vi "PrinterBarCode.vi"(8 "error in (no error)":errorcluster, 10 "PrintNum":u16 caption="列印數:", 11 "Data In":T1) -> (0 "error out":errorcluster, 3 "Data Out":T1)   [LabVIEW 2014]
uses:
  controls/Data1.ctl
  controls/Payjson.ctl
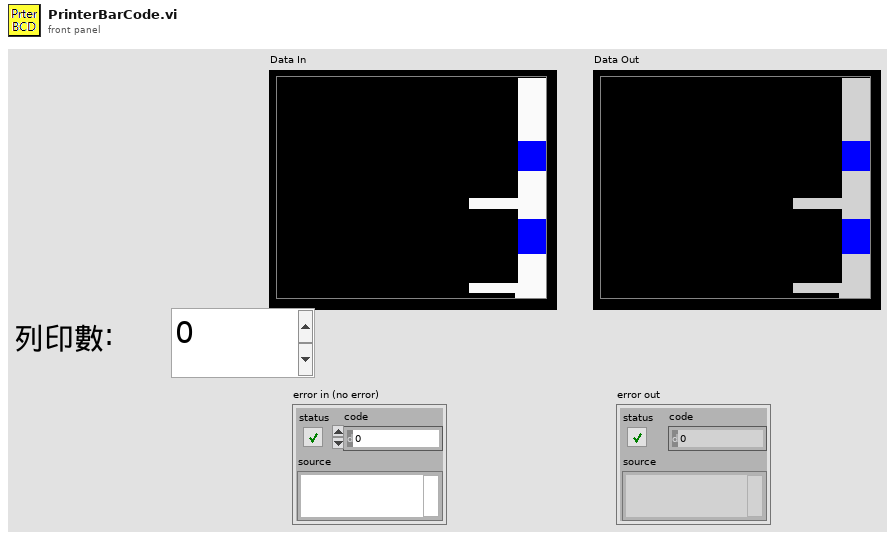
[diagram p1: front panel]
types:
  T1 = typedef "Data1.ctl" = cluster{"Date":string, "BarCode1":string, "BarCode2":string, "BarCode3":string, "Message":string, "OK Count":u16, "NG Count":u16, "Total Count":u16, "ModelData":string[][], "OK&NG":bool, "COM1":refnum<visa-resource-name>, "COM2":refnum<visa-resource-name>, "IO":i32, "Time":u32, "TCP":refnum<k5>, "TCP 2":refnum<k5>, "COM1 2":refnum<visa-resource-name>, "CheckNum":string, "BarCode1_1":string, "BarCode2_1":string, "BarCode3_1":string, "日期":string, "機種":string, "機號":string, "商品條碼1":string, "OK_1":string, "OK":string, "NG":string, "NG_1":string, "Total":string, "Total_1":string, "ClaerTime":u32, "Pjson":T2, "LotNo":string[], "CheckParsArray":string[], "BarCode4":string, "BarCode4_1":string, "商品條碼2":string, "BarCode5":string, "BarCode5_1":string, "商品條碼3":string, "ReScanNG":i32, "NGTimeCT":u32}
  T2 = typedef "Payjson.ctl" = cluster{"DEPT":string, "LINE":string, "STANO":string, "WORKNO":string, "PRODSN":string, "COMPNTID":string, "COMPNTLOT":string, "COMPNTSN":string, "USEDQTY":i16, "OPDATE":string, "OPUSER":string, "RECVDATE":string, "MMODU":string}[]
  T3 = typedef "FMT.ctl" = cluster{"formatNo":i32, "x":string, "y":string, "Is180Rotation":bool, "IsReflected":u8, "copies":u8}
  T4 = typedef "GetBIM.ctl" = cluster{"xPosition":string, "yPosition":string, "familyName":string, "emSize":sgl, "printText":string}
  T5 = typedef "QRC.ctl" = cluster{"startX":string, "startY":string, "cellSize":i32, "inoutMode":i32, "maskNumber":i32, "errorLevel":i32, "terminator":i32, "modelNumber":i32, "strData":string}
  T6 = typedef "PRT.ctl" = cluster{"quantity":i32, "cutUnit":i32, "fixedNO":i32}
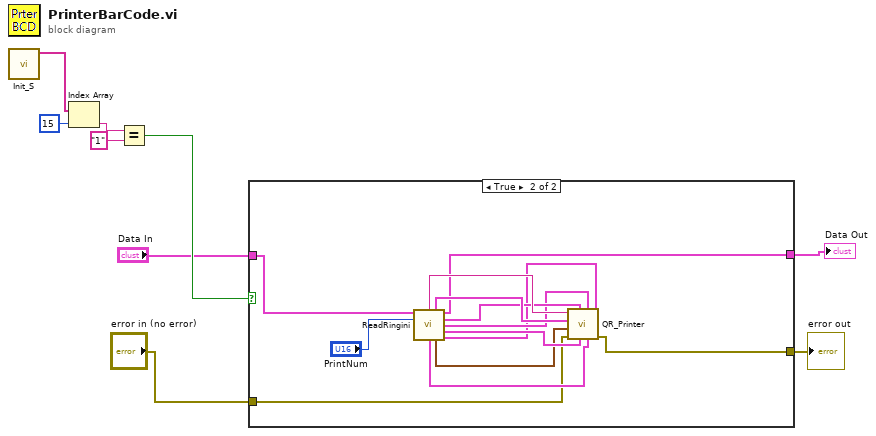
[diagram p0: block diagram]
diagram:
  n1 = call "Init_S.vi"() -> ("Path_out"=w9:string[])  [unwired: 9 in, 2 out]
  n2 = Index Array(array=w9, index=15) -> (element=w7:string)
  n3 = Equal?(x=w7, y="1") -> (x = y?=w5:bool)
  n4 = case shown="True" w5 {
    tunnel: "error in (no error)" -> [w11 w17]
    tunnel: [w11 w16] -> w3
    tunnel: "Data In" -> [w10 w15]
    tunnel: [w10 w14] -> w1
    frame False {
    }
    frame True {
      n5 = call "ReadRingini.vi"("Data In"=w15, "PrintNum"="PrintNum") -> ("PrintName"=w24:string, "FMT_out"=w23:T3, "Data Out"=w14:T1, "GetBIM_out1"=w22:T4, "GetBIM_out2"=w21:T4, "GetBIM_out3"=w20:T4, "QRC_out"=w19:T5, "PRT_out"=w18:T6, "GetBIM_out4"=w13:T4)  [unwired: 5 in]
      n6 = call "QR_Printer.vi"("GetBIM 4"=w13, "QRC"=w19, "GetBIM 2"=w21, "GetBIM 3"=w20, "GetBIM 1"=w22, "error in (no error)"=w17, "PRT"=w18, "FMT"=w23, "printName"=w24) -> ("error out"=w16:errorcluster)  [unwired: 2 in]
    }
  }
  "error out" <- w3
  "Data Out" <- w1
